vi "LIDAR to Corners.vi"(8 "Processed LIDAR":dbl[](array[numeric])=[-71.85944363103954, 13.177159590043914, 104.89019033674964, 94.69985358711568, 97.86237188872622, 105.24158125915082], 11 "Indexes":i32[](array[numeric])) -> (3 "Corner list":cluster{"X":dbl, "Y":dbl}[](array[cluster])=[{"X"=-1.0139653877484336, "Y"=0.33220956104267746}, {"X"=0.06474141933467421, "Y"=0.27652223892940664}, {"X"=4.01644189029955, "Y"=-1.0679562452867501}, {"X"=2.047093622593514, "Y"=-0.16829646561042974}, {"X"=3.9881536441467365, "Y"=-0.5507327034770187}, {"X"=1.4723244177659323, "Y"=-0.40116930197886386}])   [LabVIEW 2017]
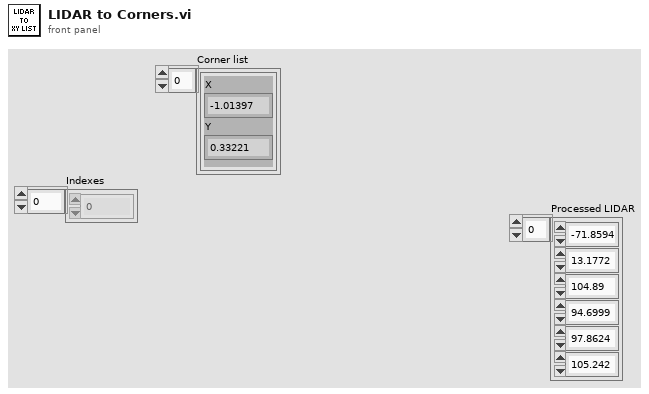
[diagram p1: front panel]
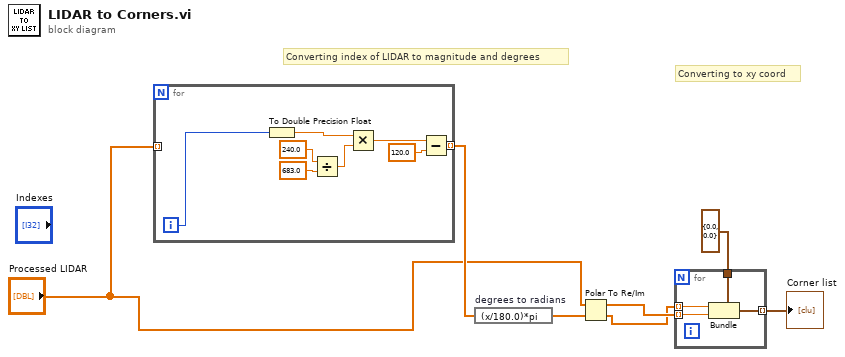
[diagram p0: block diagram]
diagram:
  # "Converting to xy coord"
  # "Converting index of LIDAR to magnitude and degrees"
  n1 = for {
    tunnel: [w9] -> w5 mode=indexing
    tunnel: "Processed LIDAR" -> [_] mode=indexing
    i -> [w8]
    n2 = To Double Precision Float(number=w8) -> (double precision float=w12:dbl)
    n3 = Divide(x=240.0, y=683.0) -> (x/y=w13:dbl)
    n4 = Multiply(x=w12, y=w13) -> (x*y=w10:dbl)
    n5 = Subtract(x=w10, y=120.0) -> (x-y=w9:dbl)
  }
  n6 = expression code="(x/180.0)*pi" "degrees to radians"(w5) -> (w4:dbl[])
  n7 = Polar To Re/Im(2:w4, 3:"Processed LIDAR") -> (0:w2:dbl[], 1:w3:dbl[])
  n8 = for {
    tunnel: w2 -> [w19] mode=indexing
    tunnel: w3 -> [w18] mode=indexing
    tunnel: cluster{"X":dbl, "Y":dbl} {"X"=0.0, "Y"=0.0} ("Point") -> [w17]
    tunnel: [w16] -> w6 mode=indexing
    n9 = Bundle(cluster=w17, "X"=w19, "Y"=w18) -> (w16:cluster{"X":dbl, "Y":dbl})
  }
  "Corner list" <- w6
